vi "Pascal Triangle.vi"() -> ()   [LabVIEW 2015]
panel:
  out "Output":string
  in  "# of Rows":i32
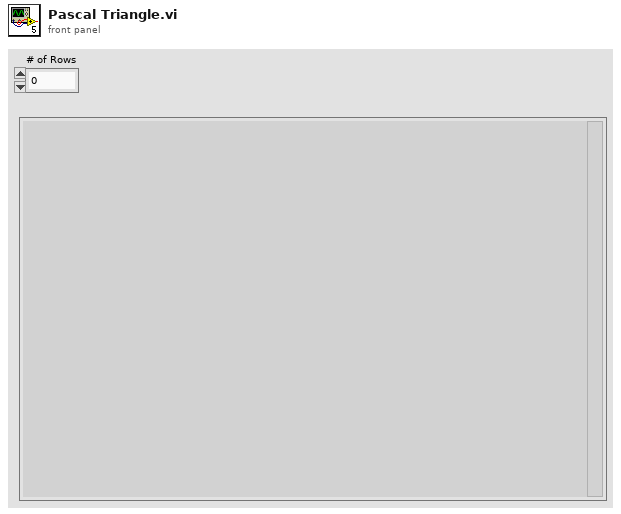
[diagram p1: front panel]
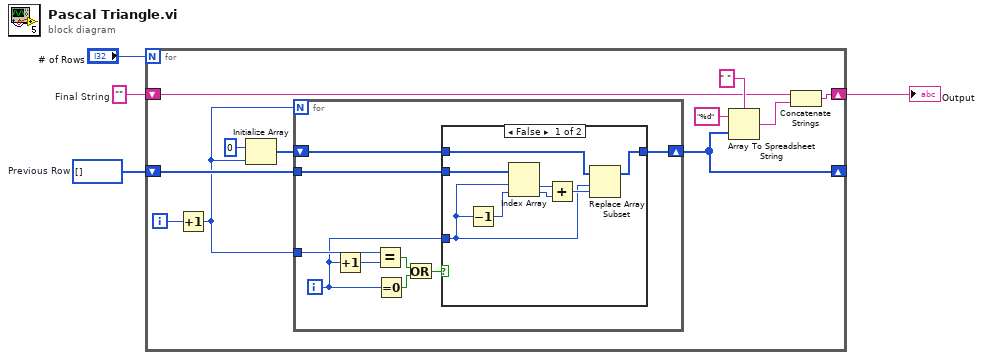
[diagram p0: block diagram]
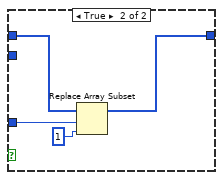
[diagram p2: hidden frame]
diagram:
  w2 = i32[] []  # Previous Row
  w3 = ""  # Final String
  n1 = for {
    N: "# of Rows" -> [_]
    shift-right: [w8] -> w1
    shift-left: w3 -> [w7]
    shift-right: [w10] -> _
    shift-left: w2 -> [w12]
    i -> [w14]
    n2 = Increment(x=w14) -> (x+1=w11:i32)
    n3 = Initialize Array(u32 0 ("element"), w11) -> (w13:u32[])
    n4 = for {
      N: w11 -> [_]
      tunnel: w11 -> [w24]
      shift-right: [w18] -> w10
      shift-left: w13 -> [w20]
      tunnel: w12 -> [w17]
      i -> [w19]
      n5 = Increment(x=w19) -> (x+1=w16:i32)
      n6 = Equal?(x=w24, y=w16) -> (x = y?=w22:bool)
      n7 = Equal To 0?(x=w19) -> (x = 0?=w23:bool)
      n8 = Or(x=w22, y=w23) -> (x .or. y?=w21:bool)
      n9 = case shown="False" w21 {
        tunnel: w20 -> [w29 w36]
        tunnel: w19 -> [w25 w35]
        tunnel: [w27 w33] -> w18
        tunnel: w17 -> [w32 _]
        frame False {
          n10 = Decrement(x=w25) -> (x-1=w26:i32)
          n11 = Index Array(array=w32, index #1=w25, index #2=w26) -> (element #1=w30:u32, element #2=w31:u32)
          n12 = Add(x=w30, y=w31) -> (x+y=w28:u32)
          n13 = Replace Array Subset(array=w29, new element=w28, index=w25) -> (w27:u32[])
        }
        frame True {
          n14 = Replace Array Subset(array=w36, new element=u32 1 ("new element/subarray"), index=w35) -> (w33:u32[])
        }
      }
    }
    n15 = Array To Spreadsheet String(delimiter (Tab)=" ", array=w10, 3:"%d" ("format string")) -> (spreadsheet string=w6:string)
    n16 = Concatenate Strings(w7, w6) -> (w8:string)
  }
  "Output" <- w1
